vi "Grid Click Callback.vi"(4 "onGridClick":refnum<user-event>, 5 "Event Data":cluster{"sender":refnum<k24>, "e":refnum<k24>}, 6 "Control Ref":refnum<k24>, 7 "Event Common Data":T1) -> ()   [LabVIEW 2024, in "SourceGrid.lvlib" / "SourceGrid.lvclass"]
uses:
  SourceGrid.lvclass
  SourceGrid.lvclass/SourceGrid.ctl
  MouseEventArgs/MouseEventArgs.lvclass
  System.Windows.Forms
  D:/git/Sourcegrid-LabVIEW/dll/SourceGrid.dll
  dll/SourceGrid.dll
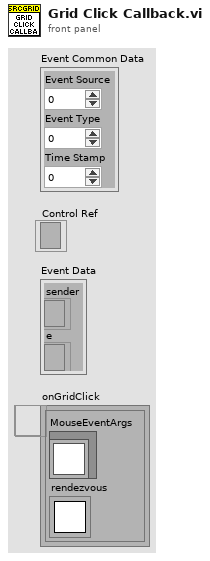
[diagram p1: front panel]
types:
  T1 = cluster{"Event Source":i32, "Event Type":u32, "Time Stamp":u32}
  T2 = typedef "Rendezvous RefNum" = refnum<k1>
  T3 = cluster{"MouseEventArgs":refnum<class "MouseEventArgs.lvclass">, "rendezvous":T2}
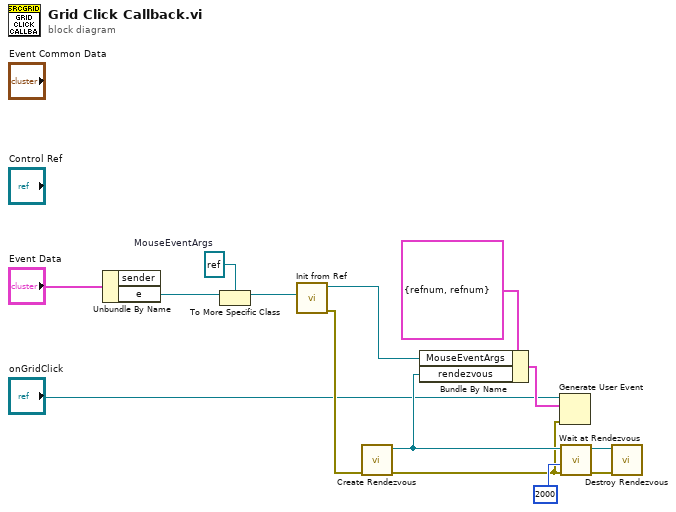
[diagram p0: block diagram]
diagram:
  w14 = refnum<k24> refnum  # MouseEventArgs
  n1 = Unbundle By Name("Event Data") -> ("e"=w13:refnum<k24>)  [unwired: 1 out]
  n2 = To More Specific Class(target class=w14, reference=w13) -> (specific class reference=w12:refnum<k24>)  [unwired: 1 in, 1 out]
  n3 = call "Init from Ref.vi"("MouseEventArgs"=w12) -> ("error out"=w4:errorcluster, "MouseEventArgs out"=w5:refnum<class "MouseEventArgs.lvclass">)  [unwired: 9 in]
  n4 = call <vilib>:"Create Rendezvous.vi"("error in (no error)"=w4) -> ("error out"=w3:errorcluster, "rendezvous"=w9:T2)  [unwired: 4 in, 1 out]
  n5 = Bundle By Name(cluster=T3 {"MouseEventArgs"=refnum, "rendezvous"=refnum} ("onClick"), "MouseEventArgs"=w5, "rendezvous"=w9) -> (w8:T3)
  n6 = Generate User Event(user event="onGridClick", event data cluster=w8, error in=w3) -> ()  [unwired: 1 in, 2 out]
  n7 = call <vilib>:"Wait at Rendezvous.vi"("error in (no error)"=w3, "ms timeout (-1)"=2000, "rendezvous"=w9) -> ("error out"=w7:errorcluster, "rendezvous out"=w6:T2)  [unwired: 2 in, 1 out]
  n8 = call <vilib>:"Destroy Rendezvous.vi"("error in (no error)"=w7, "rendezvous"=w6) -> ()  [unwired: 4 in, 2 out]
